vi "Read Base Description.vi"(11 "Mocha in":refnum<class "Soy.lvclass">) -> (2 "Description":string)   [LabVIEW 2013, in "Soy.lvclass"]
uses:
  Soy.lvclass
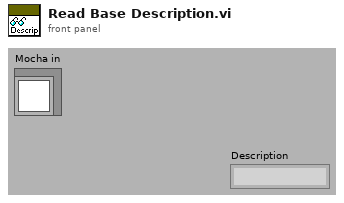
[diagram p1: front panel]
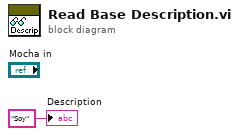
[diagram p0: block diagram]
diagram:
  "Description" <- "Soy" ("string")
